vi "pressures_sub.vi"(8 "error in (no error)":errorcluster, 11 "VISA Session In":refnum<visa-resource-name>) -> (0 "VISA Session (Dup) Gauge1":refnum<visa-resource-name>, 2 "Chamber (mbar)":dbl format="%#_3e", 3 "Back (mbar)":dbl format="%#_3e")   [LabVIEW 2018]
uses:
  Turbo Instrument Controller.llb/Type Def - Gauge Num Selection.ctl
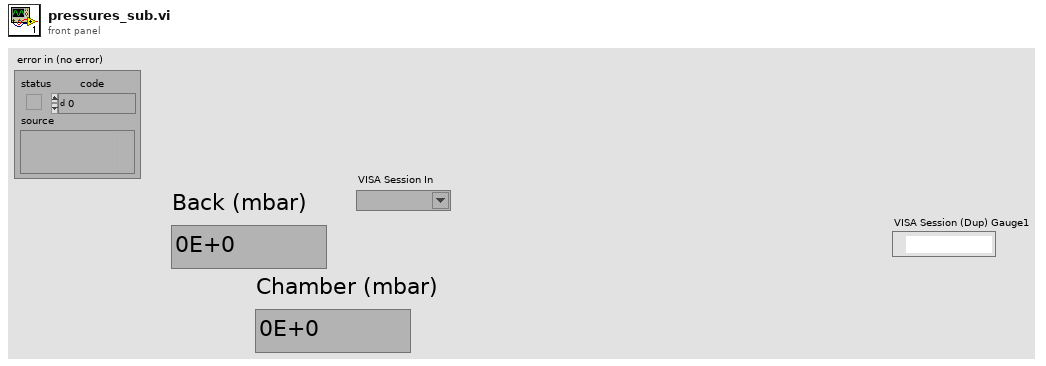
[diagram p1: front panel]
types:
  T1 = typedef "Type Def - Gauge Num Selection.ctl" = enum16{"Gauge 1", "Gauge 2", "Gauge 3", "Gauge 4", "Gauge 5", "Gauge 6"}
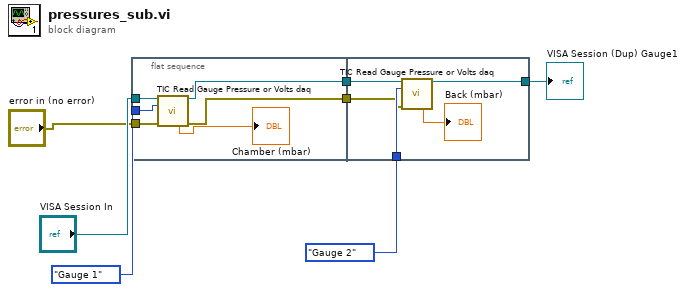
[diagram p0: block diagram]
diagram:
  n1 = flat-sequence {
    tunnel: Type_Def_-_Gauge_Num_Selection."Gauge 1" ("Gauge Number (1)") -> [w13]
    tunnel: "VISA Session In" -> [w11]
    tunnel: "error in (no error)" -> [w10]
    tunnel: [w9] -> w2
    tunnel: [w8] -> w1
    tunnel: [w17] -> w5
    tunnel: Type_Def_-_Gauge_Num_Selection."Gauge 2" ("Gauge Number (1)") -> [w18]
    tunnel: w2 -> [w15]
    tunnel: w1 -> [w14]
    frame #0 {
      n2 = call "TIC Read Gauge Pressure or Volts daq.vi"("VISA Session In"=w11, "Gauge Number (1)"=w13, "error in (no error)"=w10) -> ("VISA Session (Dup)"=w9:refnum<visa-resource-name>, "mbar"=→"Chamber (mbar)":dbl, "error out"=w8:errorcluster)  [unwired: 7 in, 3 out]
    }
    frame #1 {
      n3 = call "TIC Read Gauge Pressure or Volts daq.vi"("VISA Session In"=w15, "Gauge Number (1)"=w18, "error in (no error)"=w14) -> ("VISA Session (Dup)"=w17:refnum<visa-resource-name>, "mbar"=→"Back (mbar)":dbl)  [unwired: 7 in, 4 out]
    }
  }
  "VISA Session (Dup) Gauge1" <- w5
